vi "RW Test.vi"() -> ()   [LabVIEW 2021]
uses:
  RTFIFODouble.lvclass/RTFIFODouble.ctl
  CIFChannels/CIFChannels.lvclass/CIFChannels.ctl
  <vilib>/Utility/error.llb/Clear Errors.vi
  CIFChannels/Accessors/Write Channel State.vi
  CIFChannels/Accessors/Read Channel State.vi
  CIFChannels/Accessors/Read Direction.vi
  RTFIFODouble.lvclass
  D:/dev/CIF-LVCore/src/Channels/CIFChannels/CIFChannels.lvclass
panel:
  out "error out":errorcluster
  out "timed out? 5":bool
  out "Data 4":dbl
  out "timed out? 4":bool
  out "Data 3":dbl
  out "timed out? 3":bool
  out "Data 2":dbl
  out "timed out? 2":bool
  out "Data":dbl
  out "timed out?":bool
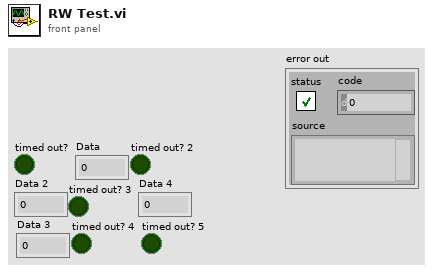
[diagram p1: front panel]
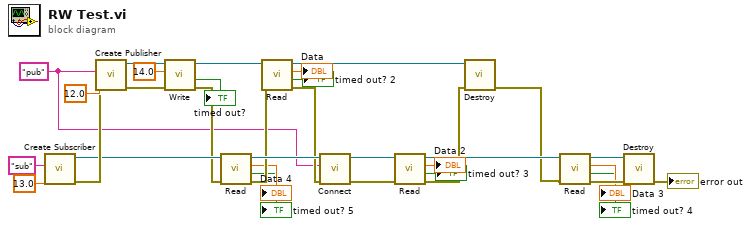
[diagram p0: block diagram]
diagram:
  w4 = "pub" ("Name")
  n1 = call "Create Subscriber.vi"("Default Value"=13.0, "Name"="sub") -> ("error out"=w28:errorcluster, "RTFIFODouble out"=w27:refnum<class "RTFIFODouble.lvclass">)  [unwired: 8 in]
  n2 = call "Create Publisher.vi"("error in (no error)"=w28, "Default Value"=12.0, "Name"=w4) -> ("error out"=w20:errorcluster, "RTFIFODouble out"=w32:refnum<class "RTFIFODouble.lvclass">)  [unwired: 7 in]
  n3 = call "Write.vi"("error in (no error)"=w20, "Data"=14.0, "RTFIFODouble in"=w32) -> ("error out"=w18:errorcluster, "timed out?"=→"timed out?":bool, "RTFIFODouble out"=w22:refnum<class "RTFIFODouble.lvclass">)  [unwired: 6 in]
  n4 = call "Read.vi"("error in (no error)"=w18, "RTFIFODouble in"=w27) -> ("error out"=w17:errorcluster, "timed out?"=→"timed out? 5":bool, "Data"=→"Data 4":dbl, "RTFIFODouble out"=w26:refnum<class "RTFIFODouble.lvclass">)  [unwired: 6 in]
  n5 = call "Read.vi"("error in (no error)"=w17, "RTFIFODouble in"=w22) -> ("error out"=w16:errorcluster, "timed out?"=→"timed out? 2":bool, "Data"=→"Data":dbl, "RTFIFODouble out"=w21:refnum<class "RTFIFODouble.lvclass">)  [unwired: 6 in]
  n6 = call-dynamic "Connect.vi"("error in (no error)"=w16, "Connection Name"=w4, "RTFIFODouble in"=w26) -> ("error out"=w15:errorcluster, "RTFIFODouble out"=w25:refnum<class "RTFIFODouble.lvclass">)  [unwired: 7 in]
  n7 = call "Read.vi"("error in (no error)"=w15, "RTFIFODouble in"=w25) -> ("error out"=w14:errorcluster, "timed out?"=→"timed out? 3":bool, "Data"=→"Data 2":dbl, "RTFIFODouble out"=w24:refnum<class "RTFIFODouble.lvclass">)  [unwired: 6 in]
  n8 = call-dynamic "Destroy.vi"("error in (no error)"=w14, "RTFIFODouble in"=w21) -> ("error out"=w13:errorcluster)  [unwired: 8 in, 1 out]
  n9 = call "Read.vi"("error in (no error)"=w13, "RTFIFODouble in"=w24) -> ("error out"=w12:errorcluster, "timed out?"=→"timed out? 4":bool, "Data"=→"Data 3":dbl, "RTFIFODouble out"=w23:refnum<class "RTFIFODouble.lvclass">)  [unwired: 6 in]
  n10 = call-dynamic "Destroy.vi"("error in (no error)"=w12, "RTFIFODouble in"=w23) -> ("error out"=→"error out":errorcluster)  [unwired: 8 in, 1 out]
